vi "Populate FP Control Refs Map.vi"(8 "error in":errorcluster, 11 "Frontpanel Ref in":refnum<vi>) -> (0 "error out":errorcluster, 2 "Control Refs":map{string, refnum<vi>}(c390), 3 "Frontpanel Ref out":refnum<vi>)   [LabVIEW 2024]
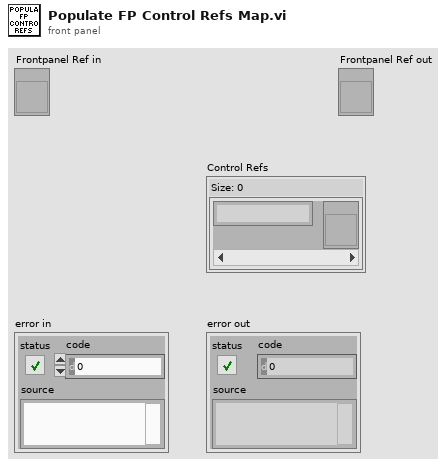
[diagram p1: front panel]
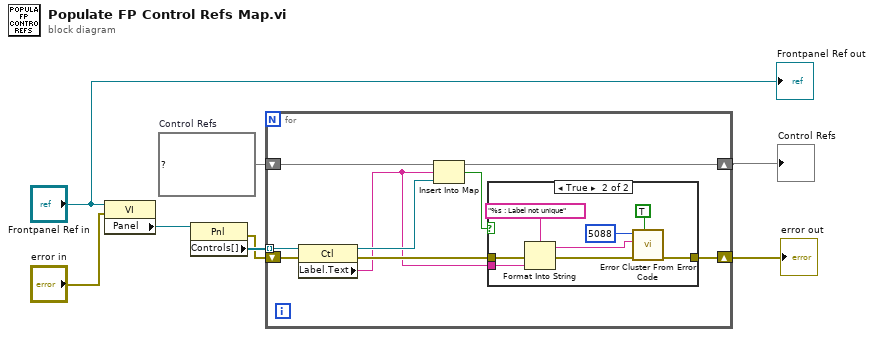
[diagram p0: block diagram]
diagram:
  w4 = map{string, refnum<vi>} {}  # Control Refs
  n1 = property class="VI"(reference="Frontpanel Ref in", error in="error in") -> ("Panel"=w8:refnum<vi>)  [unwired: 2 out]
  n2 = property class="Pnl"(reference=w8) -> (error out=w5:errorcluster, "Controls[]"=w6:refnum<vi>[])  [unwired: 1 in, 1 out]
  n3 = for {
    tunnel: w6 -> [w17] mode=indexing
    shift-right: [w13] -> w2
    shift-left: w4 -> [w16]
    shift-right: [w9] -> w3
    shift-left: w5 -> [w14]
    n4 = property class="Ctl"(reference=w17, error in=w14) -> (reference out=w15:refnum<vi>, error out=w12:errorcluster, "Label.Text"=w11:string)
    n5 = Insert Into Map(map in=w16, key=w11, value=w15) -> (map out=w13:map{string, refnum<vi>}, key already included?=w10:bool)  [unwired: 1 out]
    n6 = case shown="True" w10 {
      tunnel: w12 -> [w18 w26]
      tunnel: w11 -> [_ w24]
      tunnel: [w18 w19] -> w9
      frame False {
      }
      frame True {
        n7 = Format Into String(format string="%s : Label not unique", error in=w26, w24) -> (resulting string=w21:string, error out=w22:errorcluster)  [unwired: 1 in]
        n8 = call <vilib>:"Error Cluster From Error Code.vi"("show call chain? (False)"=TRUE, "error in (no error)"=w22, "error message (\"\")"=w21, "error code (0)"=5088) -> ("error out"=w19:errorcluster)  [unwired: 5 in]
      }
    }
  }
  "error out" <- w3
  "Control Refs" <- w2
  "Frontpanel Ref out" <- "Frontpanel Ref in"
